vi "Lidar Read.vi"(11 "I2CDevRef":T1={"DevStatus"={"status"=FALSE, "code"=0, "source"=""}, "Device Address"=0, "Handle"=0, "I2C Bus"=enum."Invalid"} {"Device Address" format="%.0x"}) -> (3 "distance (cm)":u16)   [LabVIEW 2016]
uses:
  <vilib>/Rock Robotics/WPI/I2C/WPI_I2CDevRef.ctl
  <vilib>/Rock Robotics/SystemInterfaces/i2clib/i2c_bus.ctl
panel:
  out "Data Out":u8[](array[numeric])
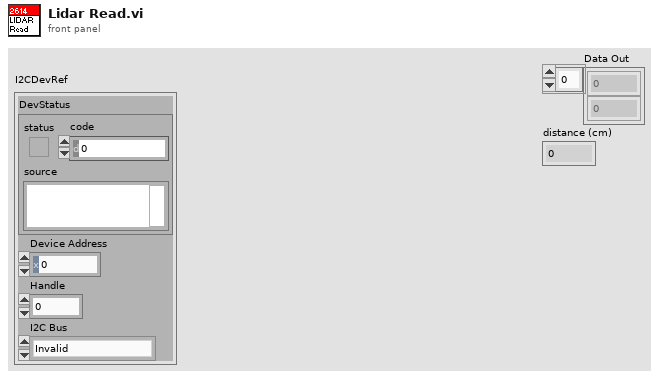
[diagram p1: front panel]
types:
  T1 = typedef "WPI_I2CDevRef.ctl" = cluster{"DevStatus":errorcluster, "Device Address":u8, "Handle":i32, "I2C Bus":T2}
  T2 = typedef "i2c_bus.ctl" = enum16{"I2C On-Board", "I2C MXP", "Invalid"}
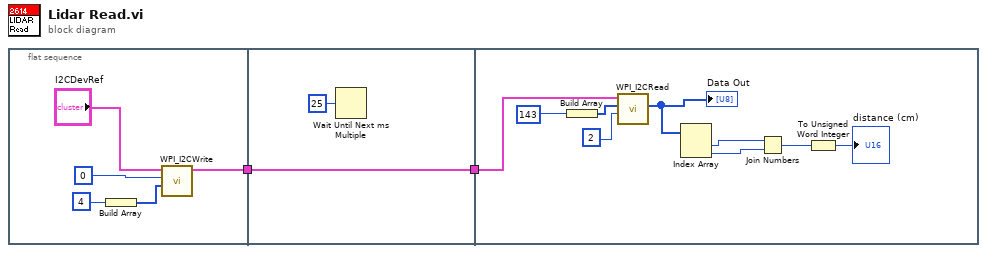
[diagram p0: block diagram]
diagram:
  n1 = flat-sequence {
    tunnel: [w6] -> w1
    tunnel: [w9] -> w2
    tunnel: w1 -> [w9]
    tunnel: w2 -> [w18]
    frame #0 {
      n2 = Build Array(u8 4) -> (w4:u8[])
      n3 = call <vilib>:"WPI_I2CWrite.vi"("I2CDataToSend"=w4, "I2CRegister"=u8 0, "I2CDevRef"="I2CDevRef") -> ("I2CDevRef"=w6:T1)  [unwired: 7 in, 1 out]
    }
    frame #1 {
      n4 = Wait Until Next ms Multiple(millisecond multiple=u32 25) -> ()  [unwired: 1 out]
    }
    frame #2 {
      n5 = Build Array(u8 143) -> (w15:u8[])
      n6 = call <vilib>:"WPI_I2CRead.vi"("I2CBytesToRead"=u8 2, "I2CRegister"=w15, "I2CDevRef"=w18) -> ("Data Out"=w14:u8[])  [unwired: 6 in, 2 out]
      "Data Out" <- w14
      n7 = Index Array(array=w14) -> (element #1=w13:u8, element #2=w12:u8)  [unwired: 2 in]
      n8 = Join Numbers(hi=w13, lo=w12) -> ((hi.lo)=w11:u16)
      n9 = To Unsigned Word Integer(number=w11) -> (unsigned 16bit integer=→"distance (cm)":u16)
    }
  }
